vi "Read Branch Rate - Returns Same Value.vi"() -> ()   [LabVIEW 2017, in "Cobertura.Tests.lvlib" / "Method.lvlib"]
uses:
  Method.lvlib
  Cobertura/Method/Method.lvclass/Method.ctl
  Cobertura/Method/Read Branch Rate.vi
  Cobertura/Method/Method.lvclass
  <vilib>/PNR/Transparent Assertions/Transparent Assertions/Transparent Assertions.lvlib
panel:
  out "error out":errorcluster
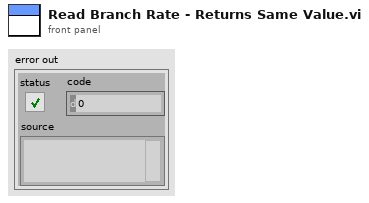
[diagram p1: front panel]
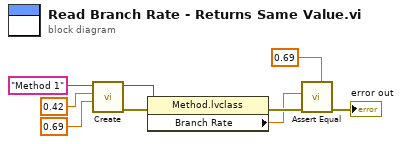
[diagram p0: block diagram]
diagram:
  n1 = call "Create.vi"("Branch Rate"=0.69, "Line Rate"=0.42, "Name"="Method 1") -> ("error out"=w6:errorcluster, "Method"=w5:refnum<class "Method.lvclass">)  [unwired: 7 in]
  n2 = property class="Method.lvclass"(reference=w5, error in=w6) -> (error out=w4:errorcluster, "Branch Rate"=w3:dbl)  [unwired: 1 out]
  n3 = call <vilib>:"Assert Equal.vi"("Expected"=0.69 ("Line Rate"), "error in (no error)"=w4, "Actual"=w3) -> ("error out"=→"error out":errorcluster)  [unwired: 8 in]
